vi "Main.vi"() -> ()   [LabVIEW 2011]
uses:
  2-Think/2 Typedefs/Which Boat.ctl
  0x2-OCU-Think Comm/0x2 Typedefs/Waypoints List.ctl
  0x2-OCU-Think Comm/0x2 Typedefs/ocuWaypoint.ctl
  0x2-OCU-Think Comm/0x2 Typedefs/waypointTypes.ctl
  2-Think/2 Typedefs/UTM Location.ctl
  0x2-OCU-Think Comm/0x2 Typedefs/Current Waypoint.ctl
  2-Think/2 Typedefs/eStopCommand.ctl
  0x2-OCU-Think Comm/0x2 Typedefs/ocuMessage.ctl
  0x2-OCU-Think Comm/0x2 Typedefs/ocuCommands.ctl
  <vilib>/Platform/TimedLoop/XDataNode/timing_clust.ctl
  <vilib>/Platform/TimedLoop/XDataNode/nitl_modes.ctl
  <vilib>/Platform/TimedLoop/XDataNode/wakeup.ctl
  <vilib>/vision/Image Controls.llb/IMAQ Image.ctl
  2-Think/2 Globals/2 Global.vi
  <vilib>/Platform/TimedLoop/XDataNode/XDataNode.xnode
  <vilib>/Platform/TimedLoop/XDataNode/XDNodeRunTimeDep.lvlib
  0x2-OCU-Think Comm/0x2 Classes/NetworkStreams/Writer/NetworkStreamWriter.lvclass
  0x2-OCU-Think Comm/0x2 Classes/NetworkStreams/Reader/NetworkStreamReader.lvclass
panel:
  out "Network \nfreq.":dbl
  in  "Which Boat Am I?":T1
  out "E-stop freq.":dbl
  out "Act freq.":dbl
  out "Sense freq.":dbl
  out "Think freq.":dbl
  in  "E-Stop":bool
  # "this is the parent VI under which \nSense Think and Act run."
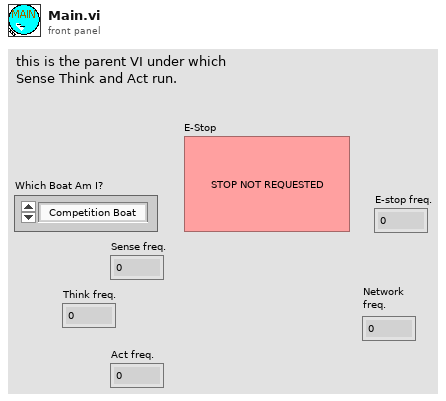
[diagram p1: front panel]
types:
  T1 = typedef "Which Boat.ctl" = enum16{"Competition Boat", "Small RC", "Simulation"}
  T2 = typedef "Waypoints List.ctl" = T3[]
  T3 = typedef "ocuWaypoint.ctl" = cluster{"Point Type":T4, "Dist/Time":dbl, "UTM Location":T5}
  T4 = typedef "waypointTypes.ctl" = enum16{"Drive", "Round Port", "Round Starboard", "Stay"}
  T5 = typedef "UTM Location.ctl" = cluster{"UTM Zone":dbl, "Hemisphere":enum16{"North", "South"}, "East":dbl, "North":dbl}
  T6 = typedef "Current Waypoint.ctl" = i32
  T7 = typedef "eStopCommand.ctl" = enum16{"Reset E-Stop", "Get E-Stop", "Set E-Stop"}
  T8 = typedef "ocuMessage.ctl" = cluster{"OCU Command":T9, "Data":variant}
  T9 = typedef "ocuCommands.ctl" = enum16{"Pass", "Send override", "Add waypoints", "Delete waypoint", "Set waypoint number", "Stop"}
  T10 = typedef "XDNodeRunTimeDep.lvlib/timing_clust.ctl" = cluster{"Expected End [f-1]":u64, "Actual End [f-1]":u64, "Finished Late? [f-1]":bool, "Expected End [i-1]":u64, "Actual End [i-1]":u64, "Finished Late? [i-1]":bool, "Expected Start [i]":u64, "Actual Start [i]":u64, "Expected Start [f]":u64, "Actual Start [f]":u64, "Source Name":string, "Structure Name":string, "Period":i64, "Deadline":i64, "Offset":i64, "Start":i64, "Priority":i32, "Timeout":i32, "Mode":T11, "Wakeup Reason":T12, "Error":errorcluster, "Source Type":string, "Secondary Source Type":string, "Global End Time":u64, "Global Start Time":u64, "Frame Duration":u64, "Iteration Duration":u64, "Assigned CPU":i32, "I/O Scan Engine Mode":u32}
  T11 = typedef "XDNodeRunTimeDep.lvlib/nitl_modes.ctl" = enum32{"No Change", "Process missed periods, maintain original phase", "Discard missed periods, maintain original phase", "Process missed periods, ignore original phase", "Discard missed periods, ignore original phase"}
  T12 = typedef "XDNodeRunTimeDep.lvlib/wakeup.ctl" = enum32{"Normal", "Aborted", "Asynchronous wakeup", "Timing source error", "Timed loop error", "Timeout"}
  T13 = typedef "IMAQ Image.ctl" = refnum<image>
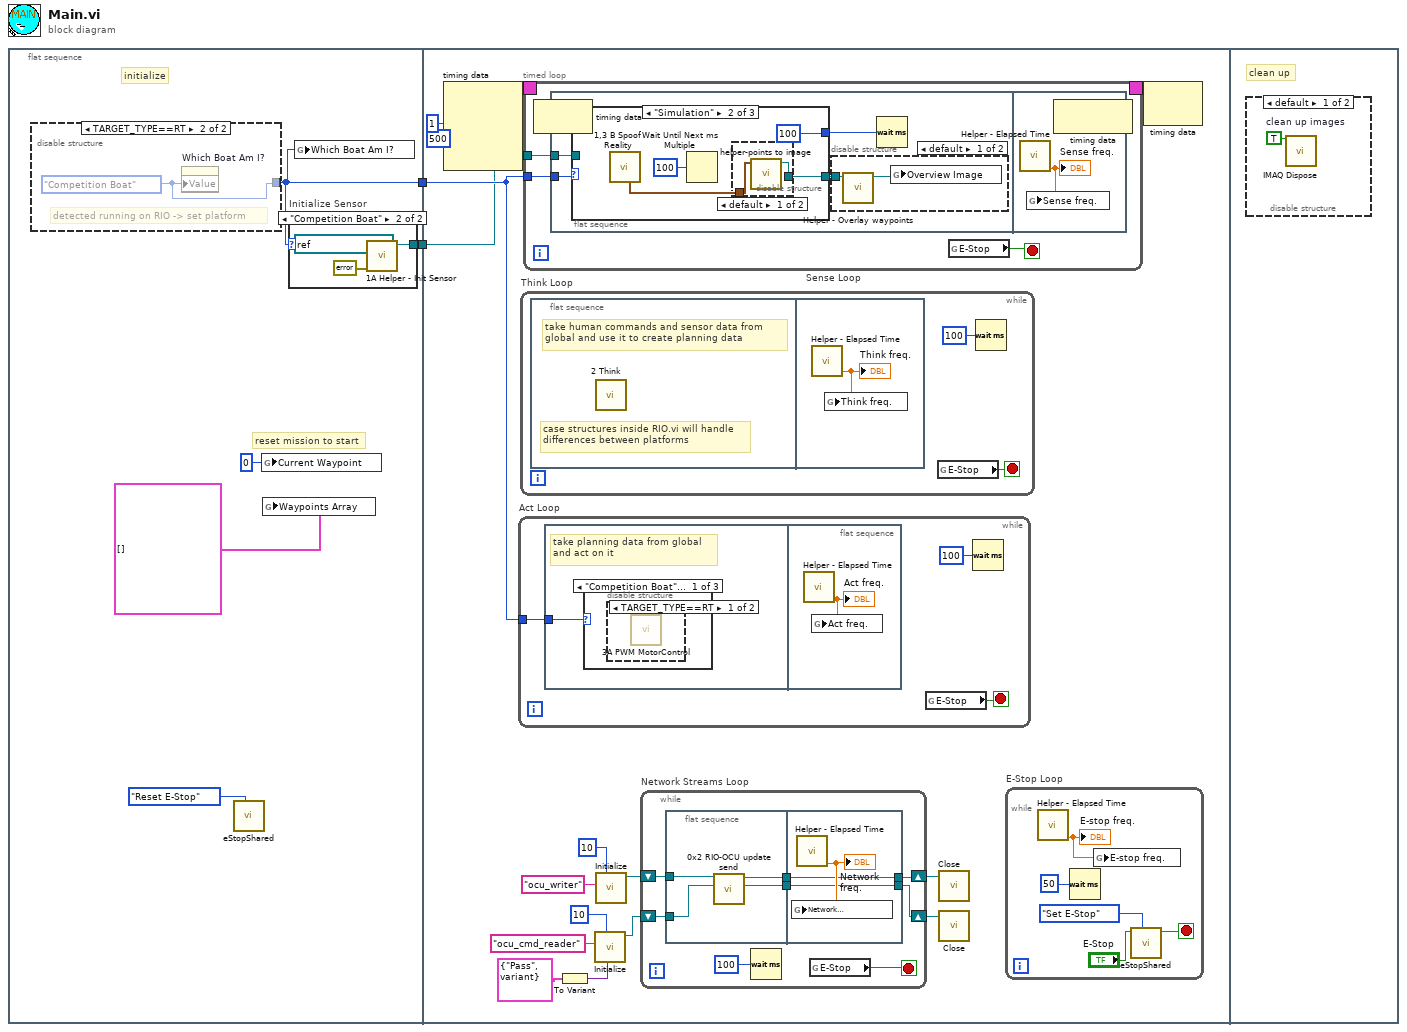
[diagram p0: block diagram]
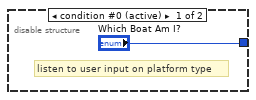
[diagram p3: hidden frame]
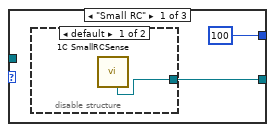
[diagram p5: hidden frame]
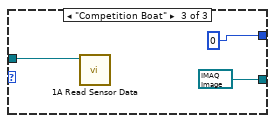
[diagram p8: hidden frame]
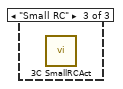
[diagram p11: hidden frame]
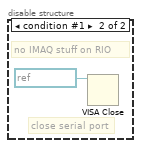
[diagram p12: hidden frame]
diagram:
  n1 = flat-sequence {
    tunnel: [w4] -> w2
    tunnel: [w5] -> w1
    tunnel: w2 -> [w28]
    tunnel: w1 -> [w27]
    frame #0 {
      # "reset mission to start"
      # "initialize"
      n2 = disable-structure shown="TARGET_TYPE==RT" {
        disable-tunnel: ["Which Boat Am I?" w12] -> w4
        frame condition #0 (active) {
          # "listen to user input on platform type"
        }
        frame condition #1 {
          w12 = Which_Boat."Competition Boat" ("Which Boat Am I?")
          # "detected running on RIO -> set platform"
          n3 = property on="Which Boat Am I?" class="Enum (strict)"("Value"=w12) -> ()  [unwired: 2 in, 2 out]
        }
      }
      n4 = call "eStopShared.vi"("Command"=eStopCommand."Reset E-Stop") -> ()  [unwired: 9 in, 2 out]
      n5 = global write "2 Global.vi" "Current Waypoint"(T6 0 ("Current Waypoint")) -> ()
      n6 = global write "2 Global.vi" "Waypoints Array"(T2 [] ("Waypoints Array")) -> ()
      n7 = case "Initialize Sensor" shown="\"Competition Boat\"" w4 {
        tunnel: [_ w8] -> w5
        frame Default {
        }
        frame "Competition Boat" {
          n8 = call "1A Helper - Init Sensor.vi"("error in (no error)"=errorcluster {"status"=FALSE, "code"=0, "source"=""}, "VISA Refnum in"=refnum<visa-resource-name> "ASRL1::INSTR" ("VISA resource name")) -> ("VISA Refnum out"=w8:refnum<visa-resource-name>)  [unwired: 8 in, 1 out]
        }
      }
      n9 = global write "2 Global.vi" "Which Boat Am I?"(w4) -> ()
    }
    frame #1 {
      n10 = node-c288(i64 1 ("Period"), 500 ("Priority")) -> (w26:T10)  [unwired: 2 in]
      n11 = while "Act Loop" {
        tunnel: w28 -> [w82]
        stop <- w83 stop-if-true
        n12 = flat-sequence {
          tunnel: w82 -> [w84]
          frame #0 {
            # "take planning data from global\nand act on it"
            n13 = case shown="\"Competition Boat\", Default" w84 {
              frame "Competition Boat", Default {
                n14 = disable-structure shown="TARGET_TYPE==RT" {
                  frame condition #0 {
                    n15 = call "3A PWM MotorControl.vi"() -> ()  [unwired: 12 in]
                  }
                  frame condition #1 (active) {
                  }
                }
              }
              frame "Simulation" {
                # "simulation Act\nis integrated with\nsimulation Think"
              }
              frame "Small RC" {
                n16 = call "3C SmallRCAct.vi"() -> ()  [unwired: 12 in]
              }
            }
          }
          frame #1 {
            n17 = call "Helper - Elapsed Time.vi"() -> ("Frequency (Hz)"=w85:dbl)  [unwired: 10 in, 1 out]
            "Act freq." <- w85
            n18 = global write "2 Global.vi" "Act freq."(w85) -> ()
          }
        }
        n19 = global read "2 Global.vi" "E-Stop"() -> (w83:bool)
        n20 = Wait (ms)(milliseconds to wait=u32 100 ("millisecond multiple")) -> ()  [unwired: 1 out]
      }
      n21 = while "Think Loop" {
        stop <- w79 stop-if-true
        n22 = flat-sequence {
          frame #0 {
            # "case structures inside RIO.vi will handle\ndifferences between platforms"
            # "take human commands and sensor data from\nglobal and use it to create planning data"
            n23 = call "2 Think.vi"() -> ()  [unwired: 12 in]
          }
          frame #1 {
            n24 = call "Helper - Elapsed Time.vi"() -> ("Frequency (Hz)"=w80:dbl)  [unwired: 10 in, 1 out]
            "Think freq." <- w80
            n25 = global write "2 Global.vi" "Think freq."(w80) -> ()
          }
        }
        n26 = global read "2 Global.vi" "E-Stop"() -> (w79:bool)
        n27 = Wait (ms)(milliseconds to wait=u32 100 ("millisecond multiple")) -> ()  [unwired: 1 out]
      }
      n28 = timed-loop "Sense Loop" {
        tunnel: w28 -> [w45]
        tunnel: w27 -> [w44]
        timing: w26 -> [_]
        timing-out: [_] -> w25
        stop <- w46 stop-if-true
        n29 = node-c288() -> ()  [unwired: 1 in, 1 out]
        n30 = flat-sequence {
          tunnel: w45 -> [w51]
          tunnel: w44 -> [w49]
          frame #0 {
            n31 = case shown="\"Simulation\"" w51 {
              tunnel: [w56 w59 T13 refnum ("Image Out")] -> w52
              tunnel: [u32 100 ("millisecond multiple") u32 100 ("millisecond multiple") u32 0 ("millisecond multiple")] -> w50
              tunnel: w49 -> [_ _ w64]
              frame "Small RC" {
                n32 = disable-structure shown="default" {
                  disable-tunnel: [w57 _] -> w56
                  frame condition #0 (active) {
                    n33 = call "1C SmallRCSense.vi"() -> ("Eye in the Sky"=w57:T13)  [unwired: 6 in, 5 out]
                  }
                  frame condition #1 {
                  }
                }
              }
              frame "Simulation" {
                n34 = call "1,3 B Spoof Reality.vi"() -> ("Boat Path"=w60:cluster{"X Position":dbl, "Y Position":dbl}[])  [unwired: 5 in, 6 out]
                n35 = Wait Until Next ms Multiple(millisecond multiple=u32 100) -> ()  [unwired: 1 out]
                n36 = disable-structure shown="default" {
                  disable-tunnel: w60 -> [w63 _]
                  disable-tunnel: [w62 _] -> w59
                  frame condition #0 (active) {
                    n37 = call "helper-points to image.vi"("Array of Points"=w63) -> ("Image Out"=w62:T13)  [unwired: 10 in]
                  }
                  frame condition #1 {
                    # "no IMAQ\non RIO"
                  }
                }
              }
              frame "Competition Boat" {
                n38 = call "1A Read Sensor Data.vi"("VISA resource name (in)"=w64) -> ()  [unwired: 9 in, 2 out]
              }
            }
            n39 = disable-structure shown="default" {
              disable-tunnel: w52 -> [w53 _]
              frame condition #0 (active) {
                n40 = call "Helper - Overlay waypoints.vi"("Img Refnum in"=w53) -> ("Img Refnum out"=w54:T13)  [unwired: 10 in]
                n41 = global write "2 Global.vi" "Overview Image"(w54) -> ()
              }
              frame condition #1 {
                # "no IMAQ stuff on RIO"
              }
            }
            n42 = Wait (ms)(milliseconds to wait=w50) -> ()  [unwired: 1 out]
          }
          frame #1 {
            n43 = call "Helper - Elapsed Time.vi"() -> ("Frequency (Hz)"=w67:dbl)  [unwired: 10 in, 1 out]
            "Sense freq." <- w67
            n44 = global write "2 Global.vi" "Sense freq."(w67) -> ()
          }
        }
        n45 = global read "2 Global.vi" "E-Stop"() -> (w46:bool)
        n46 = node-c288() -> ()  [unwired: 1 in, 1 out]
      }
      n47 = To Variant(anything=T8 {"OCU Command"=enum."Pass", "Data"=variant} ("OCU Message")) -> (Variant=w14:variant)
      n48 = call "Initialize.vi"("Default return"=w14, "writer buffer size"=10, "reader name"="ocu_cmd_reader") -> ("NetworkStreamWriter out"=w16:refnum<class "NetworkStreamReader.lvclass">)  [unwired: 7 in, 1 out]
      n49 = call "Initialize.vi"("writer buffer size"=10, "writer name"="ocu_writer") -> ("NetworkStreamWriter out"=w21:refnum<class "NetworkStreamWriter.lvclass">)  [unwired: 8 in, 1 out]
      n50 = while "Network Streams Loop" {
        shift-right: [w33] -> w20
        shift-left: w21 -> [w34]
        shift-right: [w30] -> w15
        shift-left: w16 -> [w31]
        stop <- w36 stop-if-true
        n51 = flat-sequence {
          tunnel: w34 -> [w40]
          tunnel: [w39] -> w32
          tunnel: w31 -> [w38]
          tunnel: [w37] -> w29
          tunnel: [w42] -> w33
          tunnel: w32 -> [w42]
          tunnel: [w41] -> w30
          tunnel: w29 -> [w41]
          frame #0 {
            n52 = call "0x2 RIO-OCU update send.vi"("Manual Override Reader In"=w38, "OCU Writer In"=w40) -> ("Manual Override Reader Out"=w37:refnum<class "NetworkStreamReader.lvclass">, "OCU Writer Out"=w39:refnum<class "NetworkStreamWriter.lvclass">)  [unwired: 8 in]
          }
          frame #1 {
            n53 = call "Helper - Elapsed Time.vi"() -> ("Frequency (Hz)"=w43:dbl)  [unwired: 10 in, 1 out]
            "Network \nfreq." <- w43
            n54 = global write "2 Global.vi" "Network \nfreq."(w43) -> ()
          }
        }
        n55 = Wait (ms)(milliseconds to wait=u32 100 ("millisecond multiple")) -> ()  [unwired: 1 out]
        n56 = global read "2 Global.vi" "E-Stop"() -> (w36:bool)
      }
      n57 = call "Close.vi"("NetworkStreamWriter in"=w20) -> ()  [unwired: 9 in, 2 out]
      n58 = call "Close.vi"("NetworkStreamReader in"=w15) -> ()  [unwired: 9 in, 2 out]
      n59 = while "E-Stop Loop" {
        stop <- w74 stop-if-true
        n60 = call "Helper - Elapsed Time.vi"() -> ("Frequency (Hz)"=w73:dbl)  [unwired: 10 in, 1 out]
        "E-stop freq." <- w73
        n61 = Wait (ms)(milliseconds to wait=u32 50 ("millisecond multiple")) -> ()  [unwired: 1 out]
        n62 = global write "2 Global.vi" "E-stop freq."(w73) -> ()
        n63 = call "eStopShared.vi"("Command"=eStopCommand."Set E-Stop", "E-Stop"="E-Stop") -> ("E-Stop Out"=w74:bool)  [unwired: 8 in, 1 out]
      }
      n64 = node-c288(w25) -> ()  [unwired: 1 out]
    }
    frame #2 {
      # "clean up"
      n65 = disable-structure shown="default" {
        frame condition #0 (active) {
          w86 = TRUE  # clean up images
          n66 = call "IMAQ Dispose"("All Images? (No)"=w86) -> ()  [unwired: 5 in, 1 out]
        }
        frame condition #1 {
          # "close serial port"
          # "no IMAQ stuff on RIO"
          n67 = VISA Close(VISA resource name=refnum<visa-resource-name> "COM1") -> ()  [unwired: 1 in, 1 out]
        }
      }
    }
  }
